vi "Goertz_step.vi"(0 "H_s(n-1)":dbl[](array[numeric]), 1 "H_s(n-2)":dbl[](array[numeric]), 2 "L_s(n-1)":dbl[](array[numeric]), 3 "L_s(n-2)":dbl[](array[numeric]), 4 "x(n)":dbl format="%#_13g") -> (5 "H_s(n)":dbl[](array[numeric]), 6 "L_s(n)":dbl[](array[numeric]))   [LabVIEW 2022 SP3]
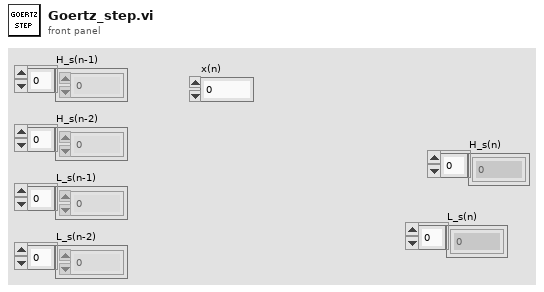
[diagram p1: front panel]
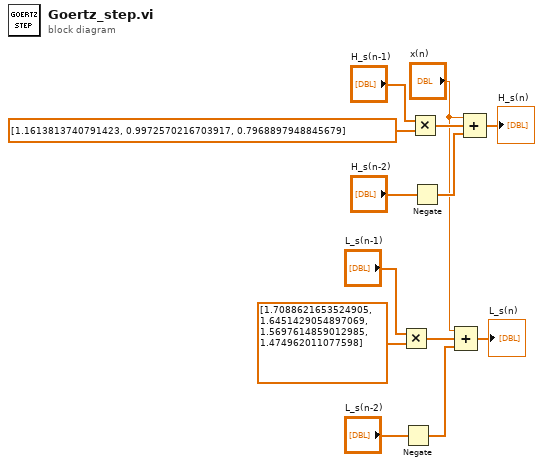
[diagram p0: block diagram]
diagram:
  n1 = Multiply(x="L_s(n-1)", y=dbl[] [1.7088621653524905, 1.6451429054897069, 1.5697614859012985, 1.474962011077598] ("2cos(L)")) -> (x*y=w3:dbl[])
  n2 = Negate(x="L_s(n-2)") -> (-x=w7:dbl[])
  n3 = Multiply(x="H_s(n-1)", y=dbl[] [1.1613813740791423, 0.9972570216703917, 0.7968897948845679] ("2cos(H)")) -> (x*y=w10:dbl[])
  n4 = Negate(x="H_s(n-2)") -> (-x=w9:dbl[])
  n5 = Compound Arithmetic op=ADD("x(n)", w3, w7) -> (→"L_s(n)":dbl[])
  n6 = Compound Arithmetic op=ADD("x(n)", w10, w9) -> (→"H_s(n)":dbl[])
